vi "catalog.wait_until_multiple_ingest_complete.vi"(6 "timeout (-1: never)":i32=-1, 8 "error in":errorcluster, 10 "datasetRid":string[](array[string]), 11 "Nominal Client":refnum<class "Nominal Client.lvclass">) -> (0 "error out":errorcluster, 3 "Nominal Client out":refnum<class "Nominal Client.lvclass">)   [LabVIEW 2018, in "Nominal Client.lvclass"]
doc: "Just for datasets"
uses:
  Nominal Client.lvclass
  Nominal Client.lvclass/Nominal Client.ctl
  catalog.get_multiple_ingest_progress_v2.vi
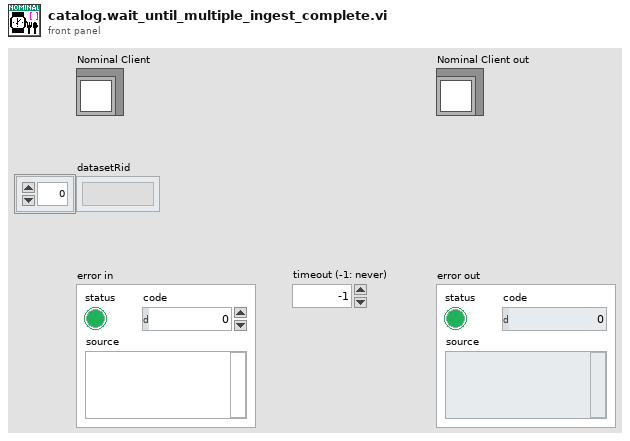
[diagram p1: front panel]
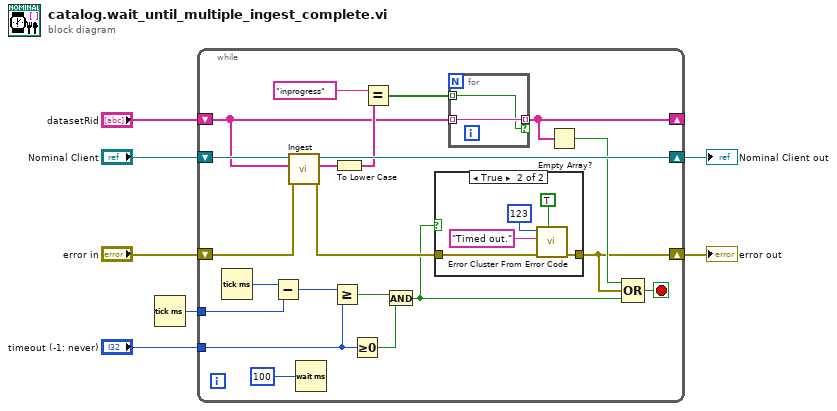
[diagram p0: block diagram]
diagram:
  n1 = Tick Count (ms)() -> (millisecond timer value=w2:u32)
  n2 = while {
    shift-right: [w26] -> w6
    shift-left: "Nominal Client" -> [w28]
    shift-right: [w13] -> w5
    shift-left: "error in" -> [w27]
    tunnel: w2 -> [w22]
    tunnel: "timeout (-1: never)" -> [w20]
    shift-right: [w8] -> _
    shift-left: "datasetRid" -> [w10]
    stop <- w25 stop-if-true
    n3 = Tick Count (ms)() -> (millisecond timer value=w23:u32)
    n4 = Subtract(x=w23, y=w22) -> (x-y=w21:u32)
    n5 = call-poly "Ingest.vi"("error in"=w27, "datasetRid[]"=w10, "Nominal Client in"=w28) -> ("error out"=w12:errorcluster, "Status"=w17:string[], "Nominal Client out"=w26:refnum<class "Nominal Client.lvclass">)  [unwired: 5 in, 1 out]
    n6 = Wait (ms)(milliseconds to wait=u32 100) -> ()  [unwired: 1 out]
    n7 = Greater Or Equal?(x=w21, y=w20) -> (x >= y?=w18:bool)
    n8 = To Lower Case(string=w17) -> (all lower case string=w16:string[])
    n9 = Greater Or Equal To 0?(x=w20) -> (x >= 0?=w19:bool)
    n10 = Equal?(x="inprogress" ("y"), y=w16) -> (x = y?=w9:bool[])
    n11 = And(x=w18, y=w19) -> (x .and. y?=w11:bool)
    n12 = case shown="True" w11 {
      tunnel: [w31 w33] -> w13
      tunnel: w12 -> [w31 w32]
      frame False {
      }
      frame True {
        n13 = call <vilib>:"Error Cluster From Error Code.vi"("show call chain? (False)"=TRUE, "error in (no error)"=w32, "error message (\"\")"="Timed out." ("error message (\"\")"), "error code (0)"=123) -> ("error out"=w33:errorcluster)  [unwired: 5 in]
      }
    }
    n14 = for {
      tunnel: w10 -> [w30] mode=indexing
      tunnel: [w30] -> w8 mode=indexing if=w29
      tunnel: w9 -> [w29] mode=indexing
    }
    n15 = Empty Array?(array=w8) -> (empty?=w14:bool)
    n16 = Compound Arithmetic op=OR(w14, w13, w11) -> (w25:bool)
  }
  "Nominal Client out" <- w6
  "error out" <- w5
